vi "Get DI Status - Multiple.vi"(0 "reference in":refnum<class "DI.lvclass">, 2 "DI Channel Numbers (Zero Based)":i32[](array[numeric]), 5 "error in (no error)":errorcluster) -> (14 "reference out":refnum<class "DI.lvclass">, 16 "DI Channel Status":bool[](array[boolean]), 19 "error out":errorcluster)   [LabVIEW 2017, in "DI.lvclass"]
uses:
  DI.lvclass
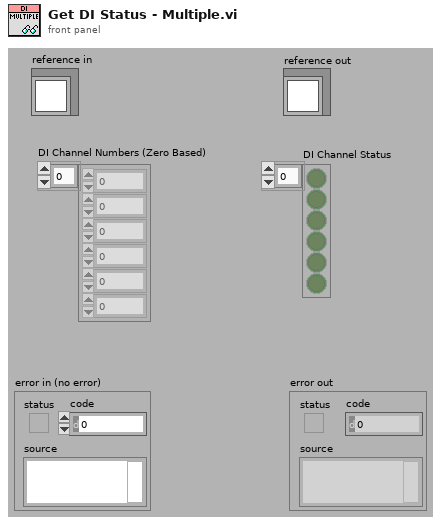
[diagram p1: front panel]
types:
  T1 = typedef "DI.lvclass/ObjectAttributes.ctl" = cluster{"DI Task":refnum<k21>, "DI Status":bool[], "DI Module Names (NI-Max Name)":string[], "Number of Channels Per DI Module":i32[], "Number of DI Modules":u32, "Number of Total DI Channels":u32, "DI On/Off Status":bool, "DO VI Reference":refnum<vi>}
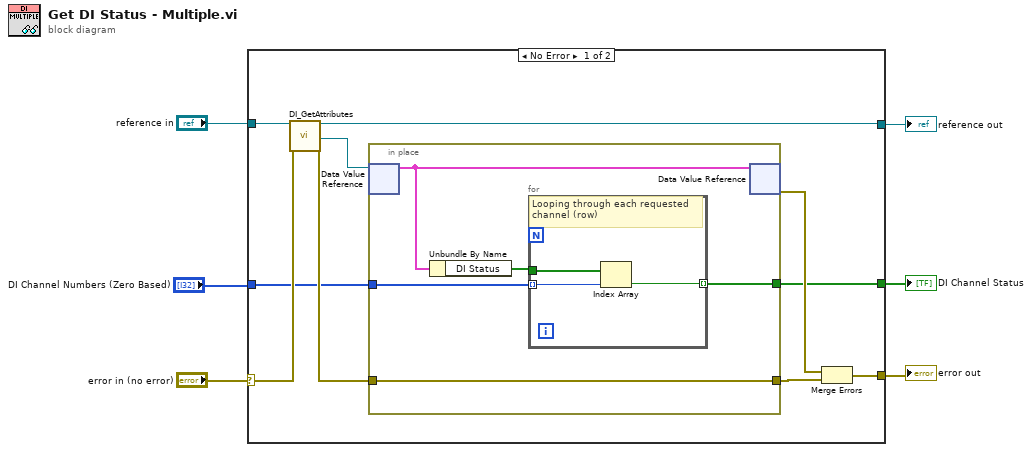
[diagram p0: block diagram]
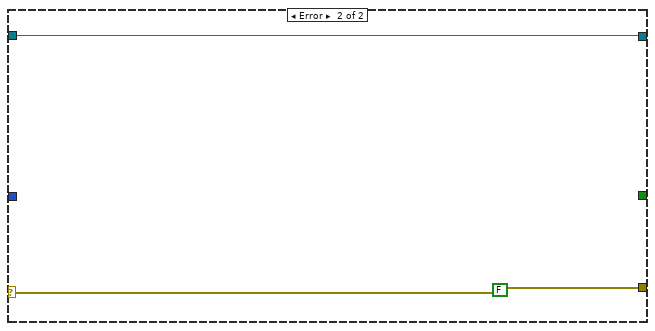
[diagram p2: hidden frame]
diagram:
  n1 = case shown="No Error" "error in (no error)" {
    selector: "error in (no error)" -> [w15 w26]
    tunnel: [w13 w26] -> w5
    tunnel: [w14 w25] -> w3
    tunnel: "reference in" -> [w16 w25]
    tunnel: "DI Channel Numbers (Zero Based)" -> [w8 _]
    tunnel: [w7 _] -> w1
    frame No Error {
      n2 = call "DI_GetAttributes.vi"("reference in"=w16, "error in (no error)"=w15) -> ("reference out"=w14:refnum<class "DI.lvclass">, "DataRef"=w12:refnum<data-value>, "error out"=w11:errorcluster)  [unwired: 14 in, 1 out]
      n3 = in-place {
        in-place-border: w11 -> [w21]
        in-place-border: [w21] -> w10
        in-place-border: w8 -> [w18]
        in-place-border: [w17] -> w7
        n4 = in-place-dvr #1(w12) -> (w20:T1)  [unwired: 1 out]
        n5 = Unbundle By Name(w20) -> ("DI Status"=w19:bool[])
        n6 = for {
          tunnel: w19 -> [w24]
          tunnel: w18 -> [w23] mode=indexing
          tunnel: [w22] -> w17 mode=indexing
          # "Looping through each requested channel (row)"
          n7 = Index Array(array=w24, index=w23) -> (element=w22:bool)
        }
        n8 = in-place-dvr #1(w20) -> (w9:errorcluster)  [unwired: 1 out]
      }
      n9 = Merge Errors(w9, w10) -> (w13:errorcluster)
    }
    frame Error {
      (unwired) FALSE
    }
  }
  "error out" <- w5
  "reference out" <- w3
  "DI Channel Status" <- w1
